vi "IMU_Viewer.vi"() -> ()   [LabVIEW 2011]
uses:
  <vilib>/Instr/_visa.llb/VISA Flush IO Buffer Mask.ctl
  <vilib>/Instr/_visa.llb/VISA Configure Serial Port (Instr).vi
  <vilib>/express/express arith-compare/Formula/XNode/ExpressFormulaBlockNode.xnode
  <vilib>/picture/3D Picture Control/NI_3D Picture Control.lvlib
panel:
  out "Kompass":dbl(knob) caption="Gauge 2" scale=0.0..360.0
  out "Magnetometer RAW":cluster{"Mx":sgl, "My":sgl, "Mz":sgl}(graph)
  out "Gyroscope RAW":cluster{"Gx":sgl, "Gy":sgl, "Gz":sgl}(graph)
  out "Lesepuffer":string
  in  "GetData":bool
  out "Acceleration RAW":cluster{"Ax":sgl, "Ay":sgl, "Az":sgl}(graph)
  out "Cluster":T1
  out "Rotation":refnum<vi>(3d-picture)
  in  "VISA resource name":refnum<visa-resource-name> caption="VISA-Ressourcenname"
  out "Vergangene Zeit":timestamp
  in  "Stopp":bool
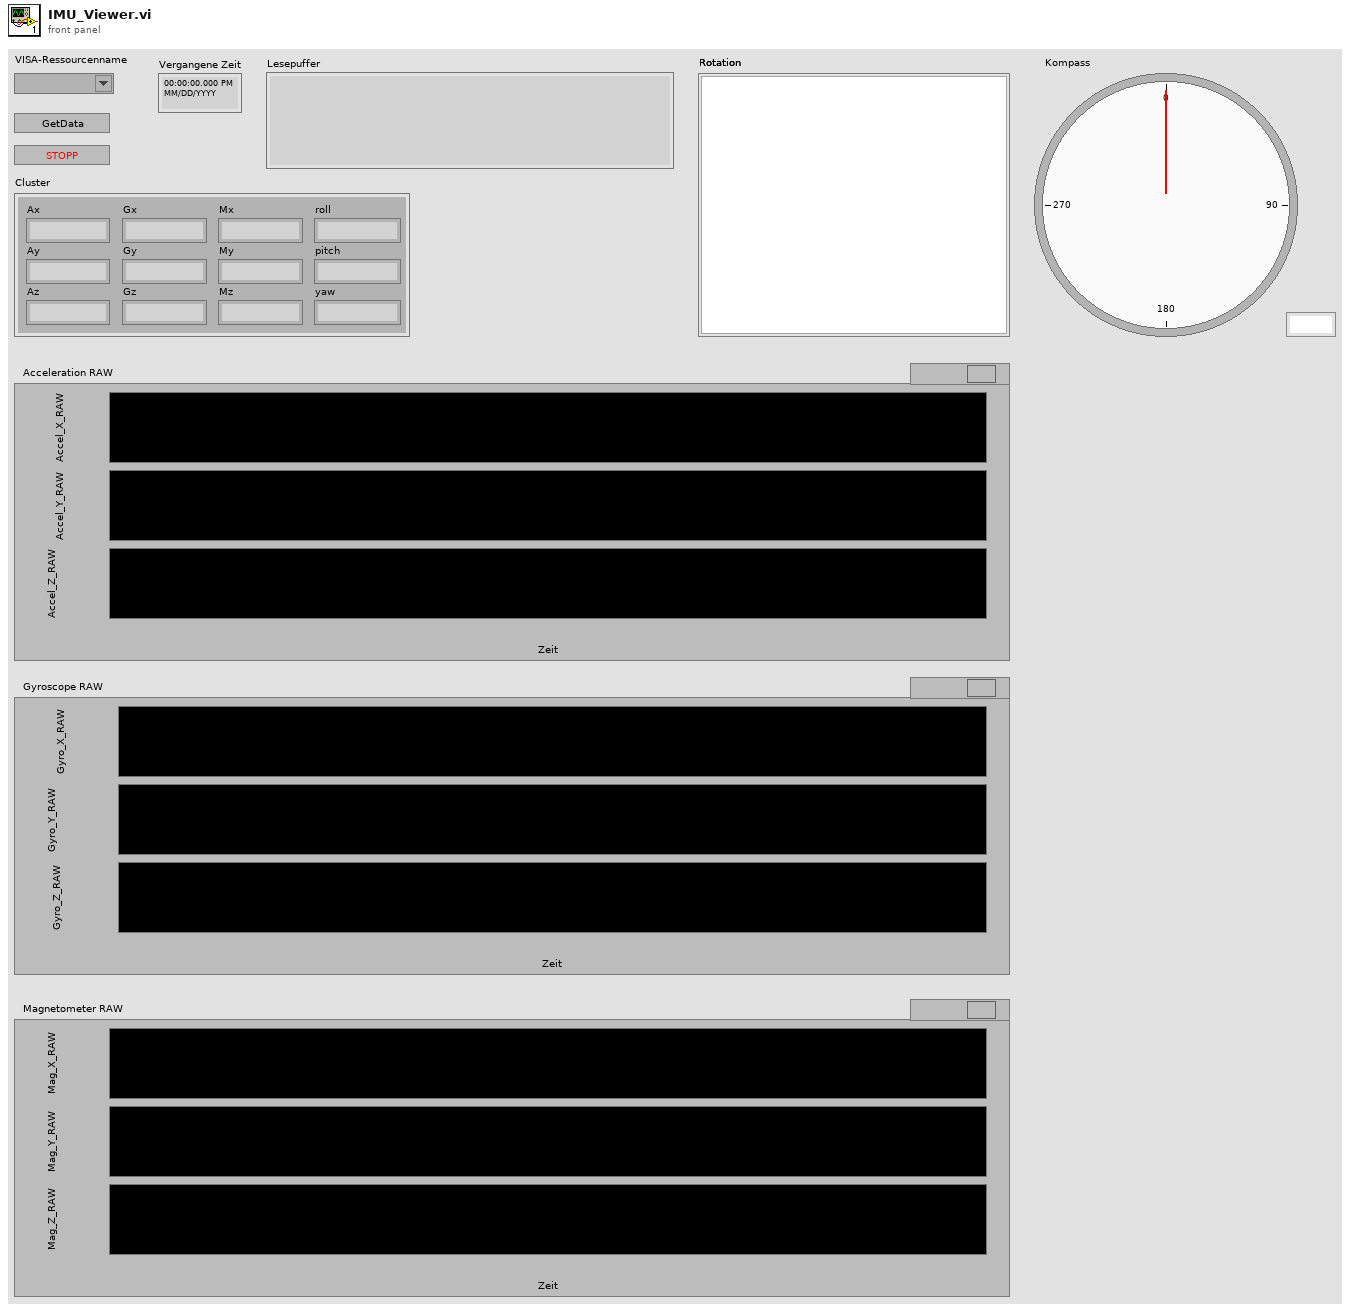
[diagram p1: front panel]
types:
  T1 = cluster{"Ax":sgl, "Ay":sgl, "Az":sgl, "Gx":sgl, "Gy":sgl, "Gz":sgl, "Mx":sgl, "My":sgl, "Mz":sgl, "roll":sgl, "pitch":sgl, "yaw":sgl}
  T2 = typedef "VISA Flush IO Buffer Mask.ctl" = u16
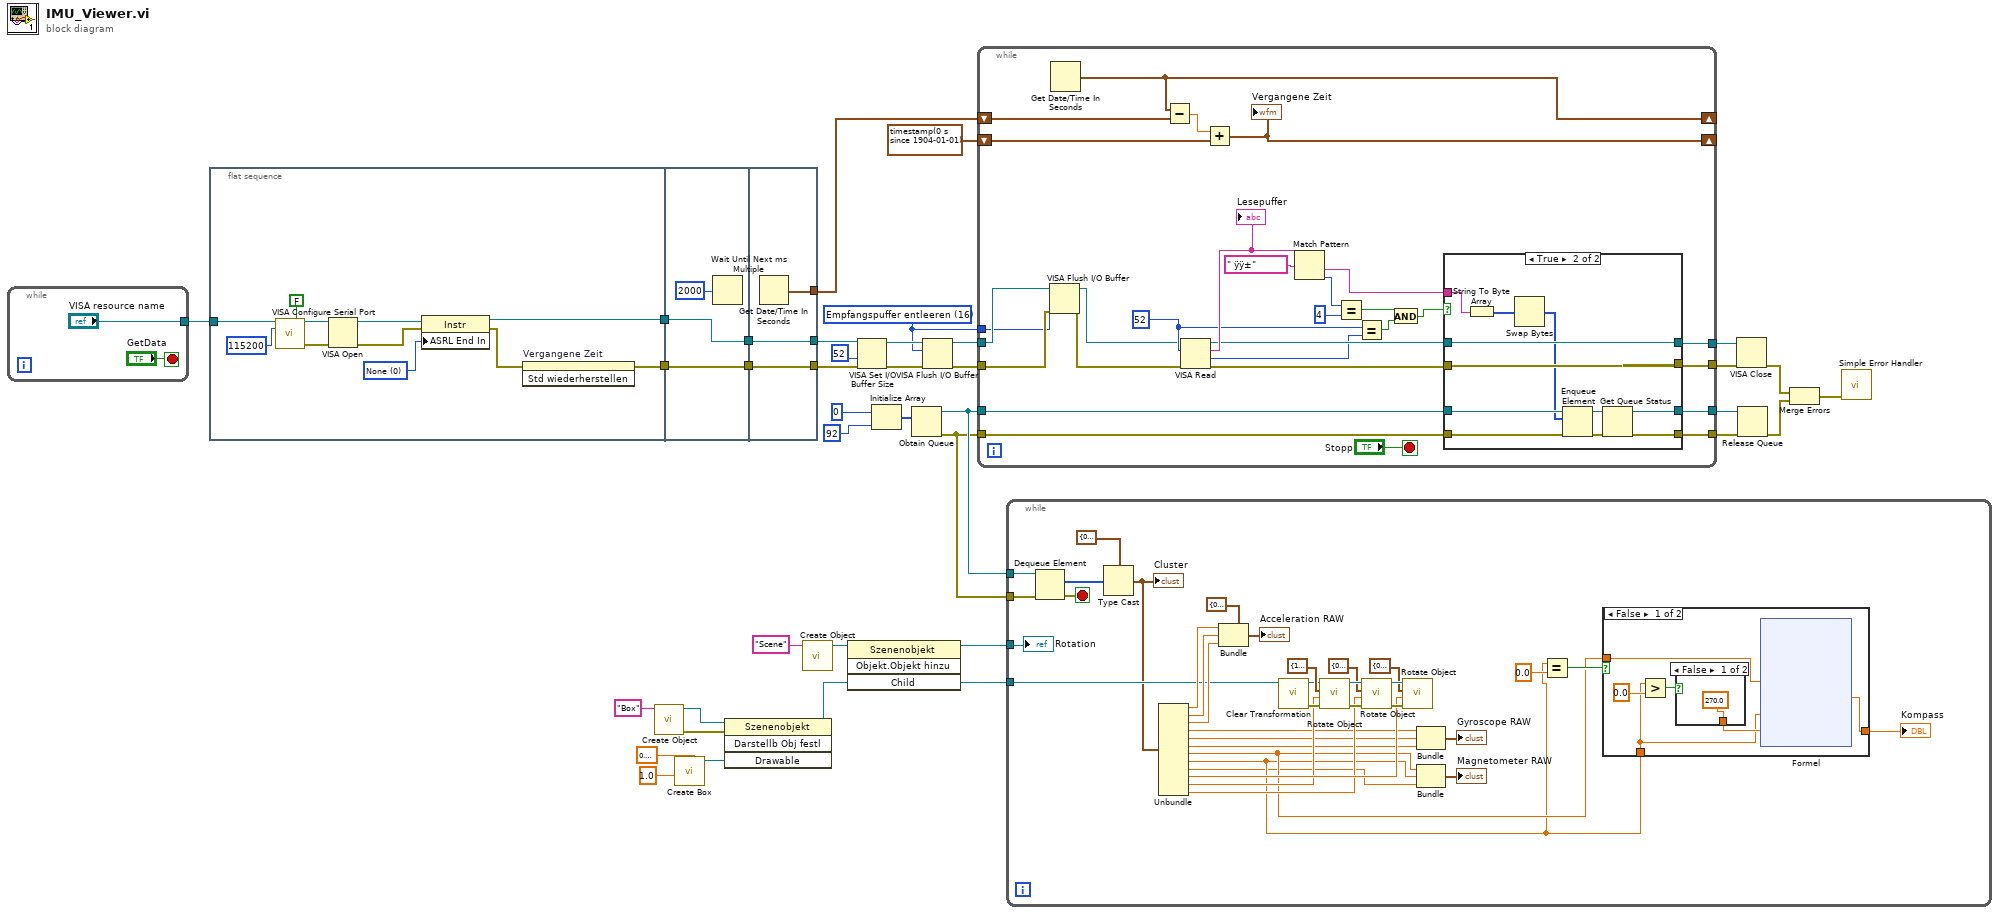
[diagram p0: block diagram]
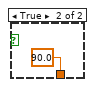
[diagram p2: hidden frame]
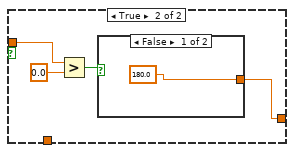
[diagram p3: hidden frame]
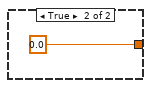
[diagram p4: hidden frame]
diagram:
  w1 = T2 16 items=["Empfangspuffer entleeren"=16, "Übertragungspuffer in Gerät schreiben"=32, "Empfangspuffer entleeren (keine I/O)"=64, "Übertragungspuffer entleeren"=128] ("Mask")
  w13 = sgl 1.0 ("Length Y")
  n1 = while {
    tunnel: ["VISA resource name"] -> w10
    stop <- "GetData" stop-if-true
  }
  n2 = flat-sequence {
    tunnel: [w42] -> w12
    tunnel: [w43] -> w11
    tunnel: w10 -> [w41]
    tunnel: [w52] -> w29
    tunnel: [w53] -> w28
    tunnel: w12 -> [w53]
    tunnel: w11 -> [w52]
    tunnel: [w57] -> w38
    tunnel: [w56] -> w16
    tunnel: w29 -> [w56]
    tunnel: [w55] -> w15
    tunnel: w28 -> [w55]
    frame #0 {
      w45 = u16 0 items=["None", "Last Bit", "TermChar"] ("Serial Settings:End Mode for Reads")
      n3 = call-poly "VISA Configure Serial Port"("VISA resource name"=w41, "Enable Termination\nChar (T)"=FALSE ("Enable Termination\nChar (T)"), "baud rate (9600)"=u32 115200) -> ("VISA resource name out"=w50:refnum<visa-resource-name>, "error out"=w51:errorcluster)  [unwired: 11 in]
      n4 = VISA Open(error in (no error)=w51, VISA resource name=w50) -> (VISA resource name=w49:refnum<visa-resource-name>, error out=w48:errorcluster)  [unwired: 3 in]
      n5 = property class="Instr"(reference=w49, error in=w48, "ASRL End In"=w45) -> (reference out=w43:refnum<visa-resource-name>, error out=w46:errorcluster)
      n6 = invoke on="Vergangene Zeit" class="AbsZeit (strikt)" method="Std wiederherstellen"(error in=w46) -> (error out=w42:errorcluster)  [unwired: 2 in, 2 out]
    }
    frame #1 {
      n7 = Wait Until Next ms Multiple(millisecond multiple=u32 2000 ("Vielfache von ms")) -> ()  [unwired: 1 out]
    }
    frame #2 {
      n8 = Get Date/Time In Seconds() -> (seconds since 1Jan1904=w57:timestamp)
    }
  }
  n9 = call <vilib>:"Create Object.vi"("Name"="Box") -> ("error out"=w22:errorcluster, "Scene:New Object"=w27:refnum<vi>)  [unwired: 9 in]
  n10 = call <vilib>:"Create Box.vi"("Length Z"=w13, "Length Y"=sgl 0.2 ("Length X"), "Length X"=w13) -> ("New Box Refnum"=w5:refnum<vi>)  [unwired: 7 in, 1 out]
  n11 = invoke class="Szenenobjekt" method="Darstellb Obj festl"(reference=w27, error in=w22, "Drawable"=w5) -> (reference out=w2:refnum<vi>)  [unwired: 1 in, 3 out]
  n12 = call <vilib>:"Create Object.vi"("Name"="Scene") -> ("Scene:New Object"=w3:refnum<vi>)  [unwired: 9 in, 1 out]
  n13 = invoke class="Szenenobjekt" method="Objekt.Objekt hinzu"(reference=w3, "Child"=w2) -> (reference out=w23:refnum<vi>, "Child"=w24:refnum<vi>)  [unwired: 2 in, 2 out]
  n14 = VISA Set I/O Buffer Size(VISA resource name=w16, size (4096)=u32 52 ("Größe (4096)"), error in (no error)=w15) -> (VISA resource name out=w6:refnum<visa-resource-name>, error out=w7:errorcluster)  [unwired: 1 in]
  n15 = Initialize Array(u8 0 ("Element"), 92 ("Dimension")) -> (w18:u8[])
  n16 = Obtain Queue(element data type=w18) -> (queue out=w26:refnum<queue>, error out=w25:errorcluster)  [unwired: 4 in, 1 out]
  n17 = VISA Flush I/O Buffer(VISA resource name=w6, mask (16)=w1, error in (no error)=w7) -> (VISA resource name out=w9:refnum<visa-resource-name>, error out=w8:errorcluster)
  n18 = while {
    shift-right: [w84] -> _
    shift-left: w38 -> [w85]
    shift-right: [w83] -> _
    shift-left: timestamp(0 s since 1904-01-01) ("seconds since 1Jan1904") -> [w69]
    tunnel: [w73] -> w36
    tunnel: [w71] -> w35
    tunnel: [w82] -> w34
    tunnel: [w81] -> w30
    tunnel: w26 -> [w79]
    tunnel: w25 -> [w80]
    tunnel: w8 -> [w60]
    tunnel: w9 -> [w62]
    tunnel: w1 -> [w58]
    stop <- "Stopp" stop-if-true
    w65 = u32 52 ("Byte-Anzahl")
    n19 = VISA Flush I/O Buffer(VISA resource name=w62, mask (16)=w58, error in (no error)=w60) -> (VISA resource name out=w61:refnum<visa-resource-name>, error out=w59:errorcluster)
    n20 = Get Date/Time In Seconds() -> (seconds since 1Jan1904=w84:timestamp)
    n21 = Subtract(x=w84, y=w85) -> (x-y=w70:dbl)
    n22 = VISA Read(VISA resource name=w61, byte count=w65, error in (no error)=w59) -> (VISA resource name out=w74:refnum<visa-resource-name>, read buffer=w77:string, return count=w64:u32, error out=w72:errorcluster)
    "Lesepuffer" <- w77
    n23 = Add(x=w70, y=w69) -> (x+y=w83:timestamp)
    "Vergangene Zeit" <- w83
    n24 = Match Pattern(string=w77, regular expression=" ÿÿ±" ("Regulärer Ausdruck")) -> (after substring=w63:string, offset past match=w76:i32)  [unwired: 1 in, 2 out]
    n25 = Equal?(x=w76, y=4) -> (x = y?=w68:bool)
    n26 = Equal?(x=w65, y=w64) -> (x = y?=w66:bool)
    n27 = And(x=w68, y=w66) -> (x .and. y?=w67:bool)
    n28 = case shown="True" w67 {
      tunnel: [w88 w95] -> w82
      tunnel: [w87 w96] -> w81
      tunnel: w80 -> [w87 w101]
      tunnel: w79 -> [w88 w100]
      tunnel: w74 -> [w90 w99]
      tunnel: [w90 w99] -> w73
      tunnel: w72 -> [w89 w98]
      tunnel: [w89 w98] -> w71
      tunnel: w63 -> [_ w93]
      frame False {
      }
      frame True {
        n29 = String To Byte Array(string=w93) -> (unsigned byte array=w92:u8[])
        n30 = Swap Bytes(anything=w92) -> (byte swapped=w91:u8[])
        n31 = Enqueue Element(queue=w100, element=w91, error in (no error)=w101) -> (queue out=w94:refnum<queue>, error out=w97:errorcluster)  [unwired: 1 in, 1 out]
        n32 = Get Queue Status(queue=w94, error in (no error)=w97) -> (queue out=w95:refnum<queue>, error out=w96:errorcluster)  [unwired: 1 in, 6 out]
      }
    }
  }
  n33 = while {
    tunnel: w25 -> [w137]
    tunnel: w26 -> [w136]
    tunnel: w24 -> [w117]
    tunnel: w23 -> [w134]
    stop <- w135 stop-if-true
    n34 = Dequeue Element(queue=w136, error in (no error)=w137) -> (element=w124:u8[], error out=w135:errorcluster)  [unwired: 1 in, 2 out]
    n35 = Type Cast(type=T1 {"Ax"=0.0, "Ay"=0.0, "Az"=0.0, "Gx"=0.0, "Gy"=0.0, "Gz"=0.0, "Mx"=0.0, "My"=0.0, "Mz"=0.0, "roll"=0.0, "pitch"=0.0, "yaw"=0.0} ("Cluster"), x=w124) -> (*(type *) &x=w112:T1)
    "Cluster" <- w112
    n36 = Unbundle(w112) -> ("Ax"=w120:sgl, "Ay"=w122:sgl, "Az"=w123:sgl, "Gx"=w107:sgl, "Gy"=w106:sgl, "Gz"=w105:sgl, "Mx"=w104:sgl, "My"=w103:sgl, "Mz"=w102:sgl, "roll"=w110:sgl, "pitch"=w109:sgl, "yaw"=w108:sgl)
    n37 = Bundle(cluster=cluster{"Ax":sgl, "Ay":sgl, "Az":sgl} {"Ax"=0.0, "Ay"=0.0, "Az"=0.0} ("Cluster"), "Ax"=w120, "Ay"=w122, "Az"=w123) -> (→"Acceleration RAW":cluster{"Ax":sgl, "Ay":sgl, "Az":sgl})
    n38 = call <vilib>:"Clear Transformation.vi"("Object Refnum In"=w117) -> ("error out"=w125:errorcluster, "Object Refnum Out"=w126:refnum<vi>)  [unwired: 9 in]
    n39 = call <vilib>:"Rotate Object.vi"("error in (no error)"=w125, "Angle"=w109, "Axis"=cluster{"X":sgl, "Y":sgl, "Z":sgl} {"X"=1.0, "Y"=0.0, "Z"=0.0}, "Scene.Object In"=w126) -> ("error out"=w128:errorcluster, "Scene.Object Out"=w133:refnum<vi>)  [unwired: 6 in]
    n40 = call <vilib>:"Rotate Object.vi"("error in (no error)"=w128, "Angle"=w108, "Axis"=cluster{"X":sgl, "Y":sgl, "Z":sgl} {"X"=0.0, "Y"=1.0, "Z"=0.0}, "Scene.Object In"=w133) -> ("error out"=w127:errorcluster, "Scene.Object Out"=w132:refnum<vi>)  [unwired: 6 in]
    n41 = call <vilib>:"Rotate Object.vi"("error in (no error)"=w127, "Angle"=w110, "Axis"=cluster{"X":sgl, "Y":sgl, "Z":sgl} {"X"=0.0, "Y"=0.0, "Z"=1.0}, "Scene.Object In"=w132) -> ()  [unwired: 6 in, 2 out]
    n42 = Bundle("Gx"=w107, "Gy"=w106, "Gz"=w105) -> (→"Gyroscope RAW":cluster{"Gx":sgl, "Gy":sgl, "Gz":sgl})  [unwired: 1 in]
    n43 = Bundle("Mx"=w104, "My"=w103, "Mz"=w102) -> (→"Magnetometer RAW":cluster{"Mx":sgl, "My":sgl, "Mz":sgl})  [unwired: 1 in]
    n44 = Equal?(x=w103, y=0.0) -> (x = y?=w116:bool)
    n45 = case shown="False" w116 {
      tunnel: w103 -> [w140 _]
      tunnel: w104 -> [w139 w159]
      tunnel: [w138 w158] -> w114
      frame False {
        n46 = Greater?(x=w140, y=0.0) -> (0:w143:bool)
        n47 = case shown="False" w143 {
          tunnel: [270.0 ("y") 90.0 ("y")] -> w141
          frame False {
          }
          frame True {
          }
        }
        n48 = xnode "Formel"("Mx"=w139, "My"=w140, "Base"=w141) -> ("Ergebnis"=w138:dbl)  [unwired: 1 in, 1 out]
      }
      frame True {
        n49 = Greater?(x=w159, y=0.0) -> (0:w161:bool)
        n50 = case shown="False" w161 {
          tunnel: [180.0 ("y") 0.0 ("y")] -> w158
          frame False {
          }
          frame True {
          }
        }
      }
    }
    "Kompass" <- w114
    "Rotation" <- w134
  }
  n51 = VISA Close(VISA resource name=w36, error in (no error)=w35) -> (error out=w33:errorcluster)
  n52 = Release Queue(queue=w34, error in (no error)=w30) -> (error out=w32:errorcluster)  [unwired: 1 in, 2 out]
  n53 = Merge Errors(w33, w32) -> (w31:errorcluster)
  n54 = call <vilib>:"Simple Error Handler.vi"("error in (no error)"=w31) -> ()  [unwired: 4 in, 5 out]
